vi "rqp_initializeManager.vi"(4 "Show in Debugger?":bool=TRUE, 6 "Message Priority":T1=enum."Normal", 7 "Caller in":refnum<class "Worker.lvclass">, 8 "error in":errorcluster, 10 "Path to JSON sequence file":path, 11 "sequenceManagerWorker in":refnum<class "sequenceManagerWorker.lvclass">) -> (0 "error out":errorcluster, 3 "dup sequenceManagerWorker out":refnum<class "sequenceManagerWorker.lvclass">, 5 "dup Caller out":refnum<class "Worker.lvclass">)   [LabVIEW 2023, in "sequenceManagerWorker.lvclass"]
doc: "This VI sends a <b>Public API Request</b> message to an MHL case of the Worker that owns this VI.\n---\nThis request loads a sequence file from disk and initializes the manager."
uses:
  sequenceManagerWorker.lvclass
  C:/Program Files (x86)/National Instruments/LabVIEW 2023/vi.lib/addons/_Workers/Library/Classes/Worker/Worker.lvclass
  <vilib>/addons/_Workers/Library/Classes/Worker/Worker.lvclass
  <vilib>/addons/_Workers/Library/Classes/Message/Priority.ctl
  <vilib>/addons/_Workers/Library/Case Label.ctl
  <vilib>/addons/_Workers/Library/Classes/Message Queue/Message Queue.lvclass
  sequenceManagerWorker.lvclass/sequenceManagerWorker.ctl
  <vilib>/addons/_Workers/Library/Workers.lvlib
  rqp_initializeManager.ctl
  <vilib>/addons/_Workers/Library/Classes/Message/Message.lvclass
panel:
  # "Connector Pane"
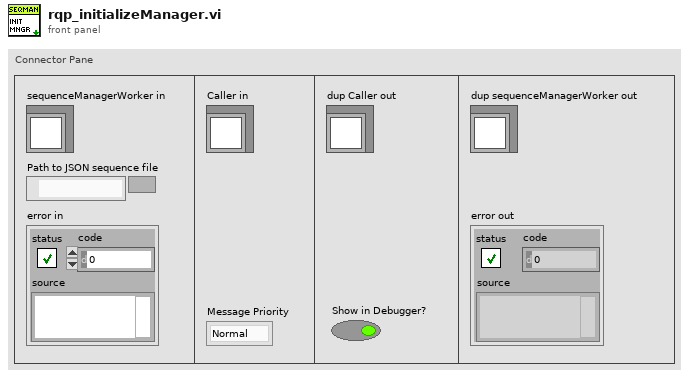
[diagram p1: front panel]
types:
  T1 = typedef "Workers.lvlib/Message.lvclass/Priority.ctl" = enum16{"Low", "Normal", "High"}
  T2 = typedef "sequenceManagerWorker.lvclass/rqp_initializeManager.ctl" = cluster{"Path to JSON sequence file":path}
  T3 = typedef "Workers.lvlib/Case Label.ctl" = string
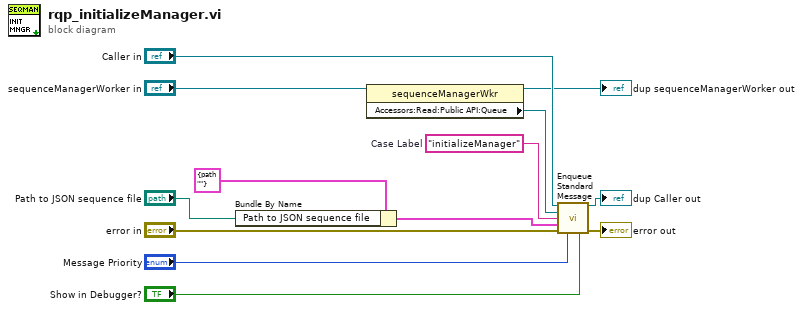
[diagram p0: block diagram]
diagram:
  w3 = T3 "initializeManager"  # Case Label
  n1 = Bundle By Name(cluster=T2 {"Path to JSON sequence file"=path ""} ("Data in"), "Path to JSON sequence file"="Path to JSON sequence file") -> (w2:T2)
  n2 = property class="sequenceManagerWkr"(reference="sequenceManagerWorker in") -> (reference out=→"dup sequenceManagerWorker out":refnum<class "sequenceManagerWorker.lvclass">, "Accessors:Read:Public API:Queue"=w4:refnum<class "Message Queue.lvclass">)  [unwired: 1 in, 1 out]
  n3 = call-dynamic "Enqueue Standard Message.vi"("Worker"="Caller in", "Message Queue"=w4, "Case Label"=w3, "Data"=w2, "error in (no error)"="error in", "Priority (Normal)"="Message Priority", "Send Message to Debugger? (T)"="Show in Debugger?") -> ("dup Worker out"=→"dup Caller out":refnum<class "Worker.lvclass">, "error out"=→"error out":errorcluster)  [unwired: 7 in]
